vi "Try Consume Regexp or Wildcard Token.vi"(10 "Name Token":T1, 11 "Pattern Parser In":T3) -> (1 "Null?":bool, 2 "Token":T1, 3 "Pattern Parser":T3)   [LabVIEW 2020, in "Stream.lvlib" / "URLPattern.lvclass"]
uses:
  URLPattern.lvclass
  Pattern Parser.ctl
  Token.ctl
  Token Type.ctl
  Pattern Part.ctl
  Pattern Part Type.ctl
  Pattern Part Modifier.ctl
  Token Type Equals.vi
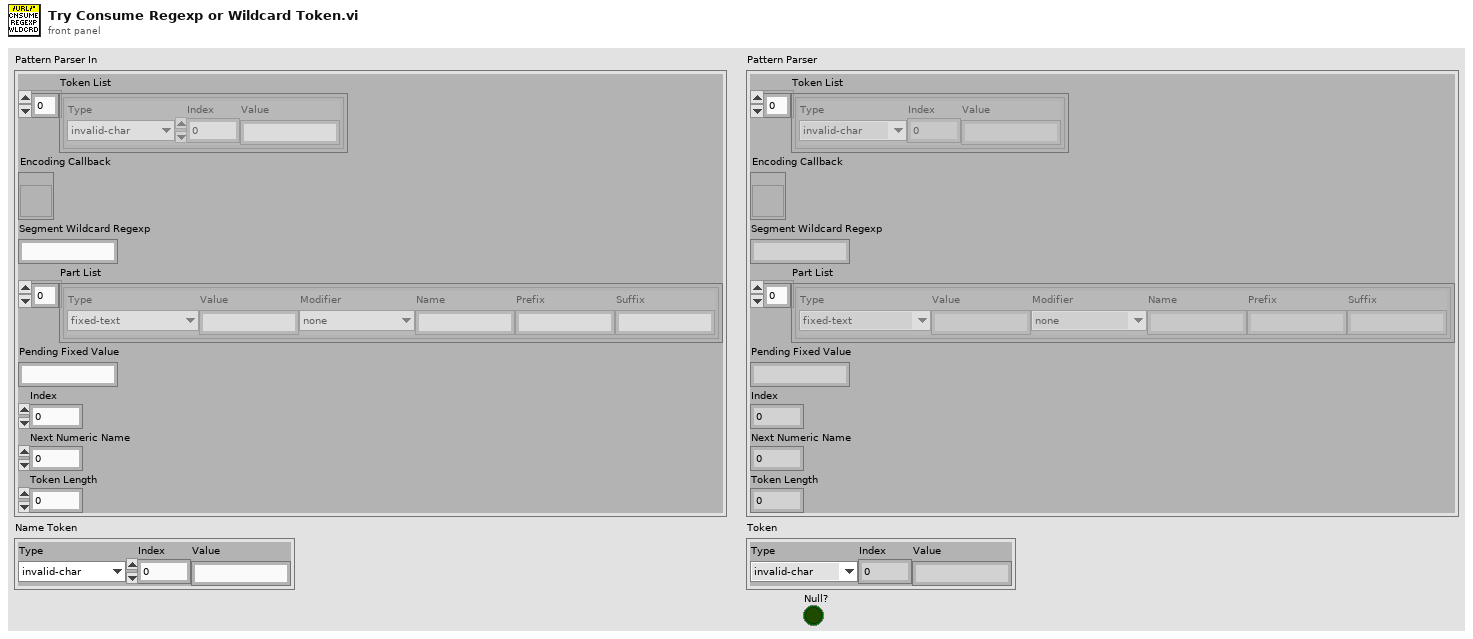
[diagram p1: front panel]
types:
  T1 = typedef "Stream.lvlib/URLPattern.lvclass/Token.ctl" = cluster{"Type":T2, "Index":i32, "Value":string}
  T2 = typedef "Stream.lvlib/URLPattern.lvclass/Token Type.ctl" = enum16{"invalid-char", "open", "close", "regexp", "name", "char", "escaped-char", "other-modifier", "asterisk", "end"}
  T3 = typedef "Stream.lvlib/URLPattern.lvclass/Pattern Parser.ctl" = cluster{"Token List":T1[], "Encoding Callback":refnum<vi>, "Segment Wildcard Regexp":string, "Part List":T4[], "Pending Fixed Value":string, "Index":i32, "Next Numeric Name":i32, "Token Length":i32}
  T4 = typedef "Stream.lvlib/URLPattern.lvclass/Pattern Part.ctl" = cluster{"Type":T5, "Value":string, "Modifier":T6, "Name":string, "Prefix":string, "Suffix":string}
  T5 = typedef "Stream.lvlib/URLPattern.lvclass/Pattern Part Type.ctl" = enum16{"fixed-text", "regexp", "segment-wildcard", "full-wildcard"}
  T6 = typedef "Stream.lvlib/URLPattern.lvclass/Pattern Part Modifier.ctl" = enum16{"none", "optional", "zero-or-more", "one-or-more"}
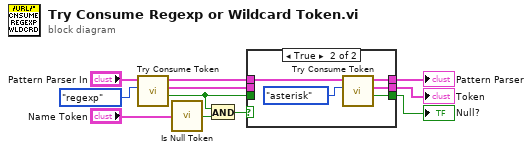
[diagram p0: block diagram]
diagram:
  n1 = call "Try Consume Token.vi"("Type"=Token_Type."regexp", "Pattern Parser In"="Pattern Parser In") -> ("Null?"=w1:bool, "Token"=w6:T1, "Pattern Parser"=w8:T3)  [unwired: 7 in]
  n2 = call "Is Null Token.vi"("Token"="Name Token") -> ("Null Token"=w9:bool)
  n3 = And(x=w1, y=w9) -> (x .and. y?=w7:bool)
  n4 = case shown="True" w7 {
    tunnel: w8 -> [w14 w19]
    tunnel: w6 -> [w13 _]
    tunnel: [w14 w17] -> w4
    tunnel: [w13 w16] -> w3
    tunnel: [w12 w15] -> w2
    tunnel: w1 -> [w12 _]
    frame False {
    }
    frame True {
      n5 = call "Try Consume Token.vi"("Type"=Token_Type."asterisk", "Pattern Parser In"=w19) -> ("Null?"=w15:bool, "Token"=w16:T1, "Pattern Parser"=w17:T3)  [unwired: 7 in]
    }
  }
  "Pattern Parser" <- w4
  "Token" <- w3
  "Null?" <- w2
